vi "Calculate Driving Direction - Kinect Mod.vi"(8 "error in (no error)":errorcluster, 9 "reader endpoint":refnum<k21>, 10 "obstacle angles (rad)":dbl[](array[numeric]), 11 "obstacle distances (m)":dbl[](array[numeric])) -> (0 "error out":errorcluster, 1 "Reader endpoint out":refnum<k21>, 3 "steering frame velocity":dbl[](array[numeric]))   [LabVIEW 2010]
doc: "Calculates the velocity vector of the robot required to avoid obstacles, based on the scanned data."
uses:
  <vilib>/robotics/Obstacle Avoidance/Simple Vector Field Histogram/NI_Robotics_Simple Vector Field Histogram.lvlib
  <vilib>/robotics/Obstacle Avoidance/Simple Vector Field Histogram/Panic Range.ctl
  <vilib>/Utility/AngleManip/NI_AngleManipulation.lvlib
  <vilib>/Utility/AngleManip/Degrees to Radians (Scalar DBL).vi
  <vilib>/robotics/Obstacle Avoidance/Simple Vector Field Histogram/Gap Description.ctl
  <vilib>/robotics/Obstacle Avoidance/Simple Vector Field Histogram/Obstacle Description.ctl
  Kinect VIs/Kinect Heading Data.ctl
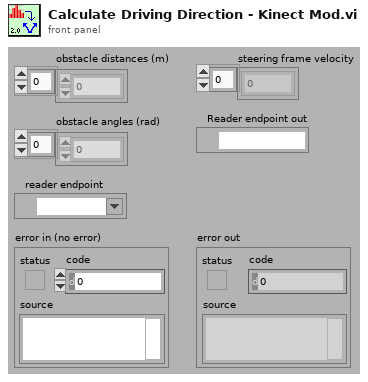
[diagram p1: front panel]
types:
  T1 = typedef "NI_Robotics_Simple Vector Field Histogram.lvlib/Panic Range.ctl" = cluster{"panic threshold distance (0)":dbl, "panic threshold angle (0)":dbl}
  T2 = typedef "Kinect Heading Data.ctl" = cluster{"largest gap":T3, "nearest obstacle":T4, "obstacle within panic range":bool}
  T3 = typedef "NI_Robotics_Simple Vector Field Histogram.lvlib/Gap Description.ctl" = cluster{"angle to gap":dbl, "size of gap":dbl}
  T4 = typedef "NI_Robotics_Simple Vector Field Histogram.lvlib/Obstacle Description.ctl" = cluster{"angle to obstacle":dbl, "distance to obstacle":dbl}
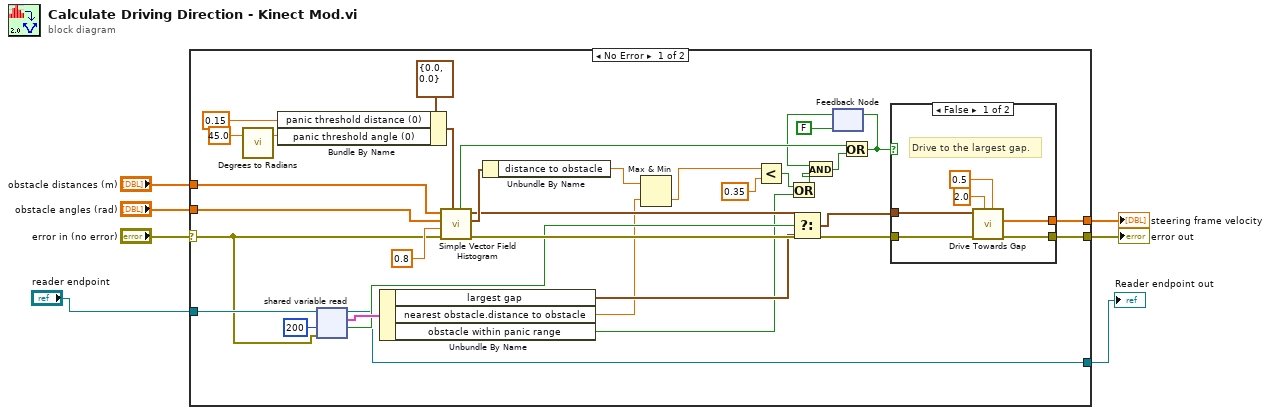
[diagram p0: block diagram]
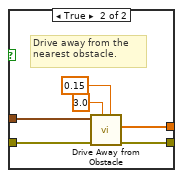
[diagram p2: hidden frame]
diagram:
  n1 = case shown="No Error" "error in (no error)" {
    selector: "error in (no error)" -> [w9 w54]
    tunnel: [w26 w54] -> w7
    tunnel: "obstacle distances (m)" -> [w25 _]
    tunnel: "obstacle angles (rad)" -> [w24 _]
    tunnel: [w23 _] -> w3
    tunnel: "reader endpoint" -> [w22 w53]
    tunnel: [w8 w53] -> w1
    frame No Error {
      n2 = call-poly <vilib>:"Degrees to Radians.vi"("angle (deg)"=45.0 ("panic threshold angle (rad)")) -> ("angle (rad)"=w40:dbl)  [unwired: 2 in]
      n3 = Bundle By Name(cluster=T1 {"panic threshold distance (0)"=0.0, "panic threshold angle (0)"=0.0} ("panic range"), "panic threshold distance (0)"=0.15 ("panic threshold distance (m)"), "panic threshold angle (0)"=w40) -> (w30:T1)
      n4 = shared-variable-read(w22, w9, 200 ("timeout ms (-1)")) -> (w8:refnum<k21>, w19:bool, w20:T2)  [unwired: 1 out]
      n5 = Unbundle By Name(w20) -> ("largest gap"=w17:T3, "nearest obstacle.distance to obstacle"=w14:dbl, "obstacle within panic range"=w11:bool)
      n6 = call <vilib>:"Simple Vector Field Histogram.vi"("panic range"=w30, "error in (no error)"=w9, "distance threshold"=0.8 ("distance threshold (m)"), "direction angles"=w24, "distances"=w25) -> ("error out"=w27:errorcluster, "nearest obstacle"=w32:T4, "largest gap"=w18:T3, "obstacle within panic range"=w35:bool)  [unwired: 2 in, 1 out]
      n7 = Unbundle By Name(w32) -> ("distance to obstacle"=w15:dbl)
      n8 = Max & Min(x=w15, y=w14) -> (min(x,y)=w13:dbl)  [unwired: 1 out]
      n9 = Less?(x=w13, y=0.35) -> (x < y?=w12:bool)
      n10 = Or(x=w12, y=w11) -> (x .or. y?=w10:bool)
      n11 = Select(t=w18, s=w19, f=w17) -> (s? t:f=w16:T3)
      n12 = feedback #1(FALSE ("obstacle within panic range")) -> (w34:bool)
      n13 = And(x=w34, y=w10) -> (x .and. y?=w36:bool)
      n14 = Or(x=w35, y=w36) -> (x .or. y?=w38:bool)
      n15 = feedback-in #1(w38) -> ()
      n16 = case shown="False" w38 {
        tunnel: w16 -> [w45 w50]
        tunnel: w27 -> [w46 w52]
        tunnel: [w44 w51] -> w26
        tunnel: [w43 w49] -> w23
        frame False {
          # "Drive to the largest gap."
          n17 = call "Drive Towards Gap.vi"("max forward velocity (m/s)"=0.5, "max angular velocity (rad/s)"=2.0, "error in (no error)"=w46, "gap"=w45) -> ("error out"=w44:errorcluster, "steering frame velocity"=w43:dbl[])  [unwired: 6 in]
        }
        frame True {
          # "Drive away from the nearest obstacle."
          n18 = call "Drive Away from Obstacle.vi"("max reverse velocity (m/s)"=0.15, "max angular velocity (rad/s)"=3.0, "error in (no error)"=w52, "gap"=w50) -> ("error out"=w51:errorcluster, "steering frame velocity"=w49:dbl[])  [unwired: 6 in]
        }
      }
    }
    frame Error {
    }
  }
  "error out" <- w7
  "steering frame velocity" <- w3
  "Reader endpoint out" <- w1
